vi "Add Item to Listbox.vi"(8 "error in (no error)":errorcluster, 10 "Item":string[](array[string]), 11 "MulticolumnListbox in":refnum<vi>) -> (0 "error out":errorcluster)   [LabVIEW 2015, in "Diagnostics Addon System Explorer.lvlib"]
uses:
  Diagnostics Addon System Explorer.lvlib
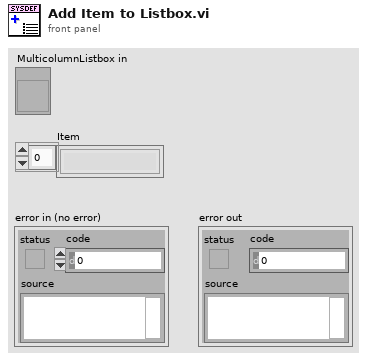
[diagram p1: front panel]
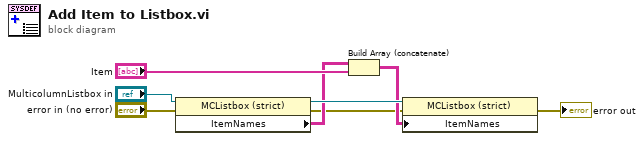
[diagram p0: block diagram]
diagram:
  n1 = property class="MCListbox (strict)"(reference="MulticolumnListbox in", error in="error in (no error)") -> (reference out=w7:refnum<vi>, error out=w3:errorcluster, "ItemNames"=w5:string[][])
  n2 = Build Array (concatenate)(w5, "Item") -> (w6:string[][])
  n3 = property class="MCListbox (strict)"(reference=w7, error in=w3, "ItemNames"=w6) -> (error out=→"error out":errorcluster)  [unwired: 1 out]
